vi "OFBS_train_kNN.vi"(6 "Train Data":T4, 8 "error in (no error)":errorcluster, 9 "k":i32, 10 "Parameters":i32[](array[numeric]), 11 "OFBS class in":refnum<class "OptFreqBandsSearch.lvclass">) -> (0 "error out":errorcluster, 1 "Training Results":T2[](array[typedef]) {"Standard Deviation" format="%.2f"}, 2 "Classifier Session (out)":T3, 3 "OFBS class out":refnum<class "OptFreqBandsSearch.lvclass">)   [LabVIEW 2016, in "Optimal Frequency Bands Search.lvlib" / "OptFreqBandsSearch.lvclass"]
doc: "Метод, реализующий построение классификатора на основе многослойного персептрона. Для обучения классификатора используются обучающие данные."
uses:
  OptFreqBandsSearch.lvclass
  OFBS_DataTypes.ctl
  <vilib>/vision/Classification.llb/IMAQ Classifier Session.ctl
  <vilib>/vision/Classification.llb/IMAQ Classifier Nearest Neighbor Training Results.ctl
  <vilib>/vision/Classification.llb/IMAQ Classifier Nearest Neighbor options.ctl
  OptFreqBandsSearch.lvclass/OptFreqBandsSearch.ctl
  Optimal Frequency Bands Search.lvlib
  <vilib>/vision/NI_Vision_Development_Module.lvlib
panel:
  in  "Nearest Neighbor Options":T1={"Method"=1, "Metric"=2, "k"=3} {"Method" items=["Nearest Neighbor", "K Nearest Neighbor", "Minimum Mean Distance"]; "Metric" items=["Maximum", "Sum", "Euclidean"]; "k" min=3}
  # "This VI is a part of BCI Design library, http://www.ru-bci.org \nCopyright © 2020, Sotnikov Peter, All rights reserved. License: CC BY-NC 4.0"
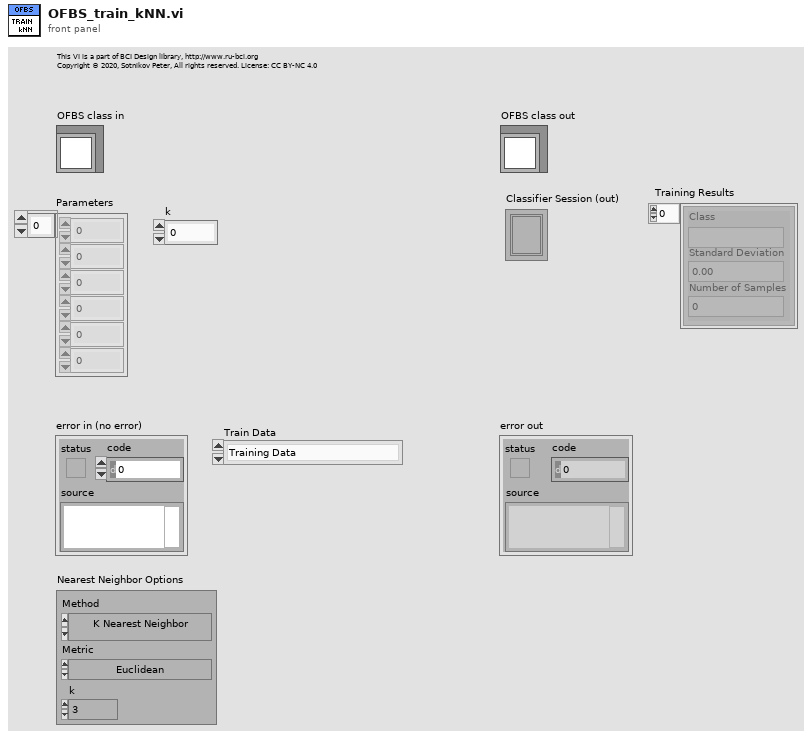
[diagram p1: front panel]
types:
  T1 = typedef "IMAQ Classifier Nearest Neighbor options.ctl" = cluster{"Method":i32, "Metric":i32, "k":i32}
  T2 = typedef "IMAQ Classifier Nearest Neighbor Training Results.ctl" = cluster{"Class":string, "Standard Deviation":sgl, "Number of Samples":i32}
  T3 = typedef "IMAQ Classifier Session.ctl" = refnum<k1>
  T4 = typedef "Optimal Frequency Bands Search.lvlib/OFBS_DataTypes.ctl" = enum16{"Training Data", "Test Data", "Training Data (cross-check)", "Test Data (cross-check)"}
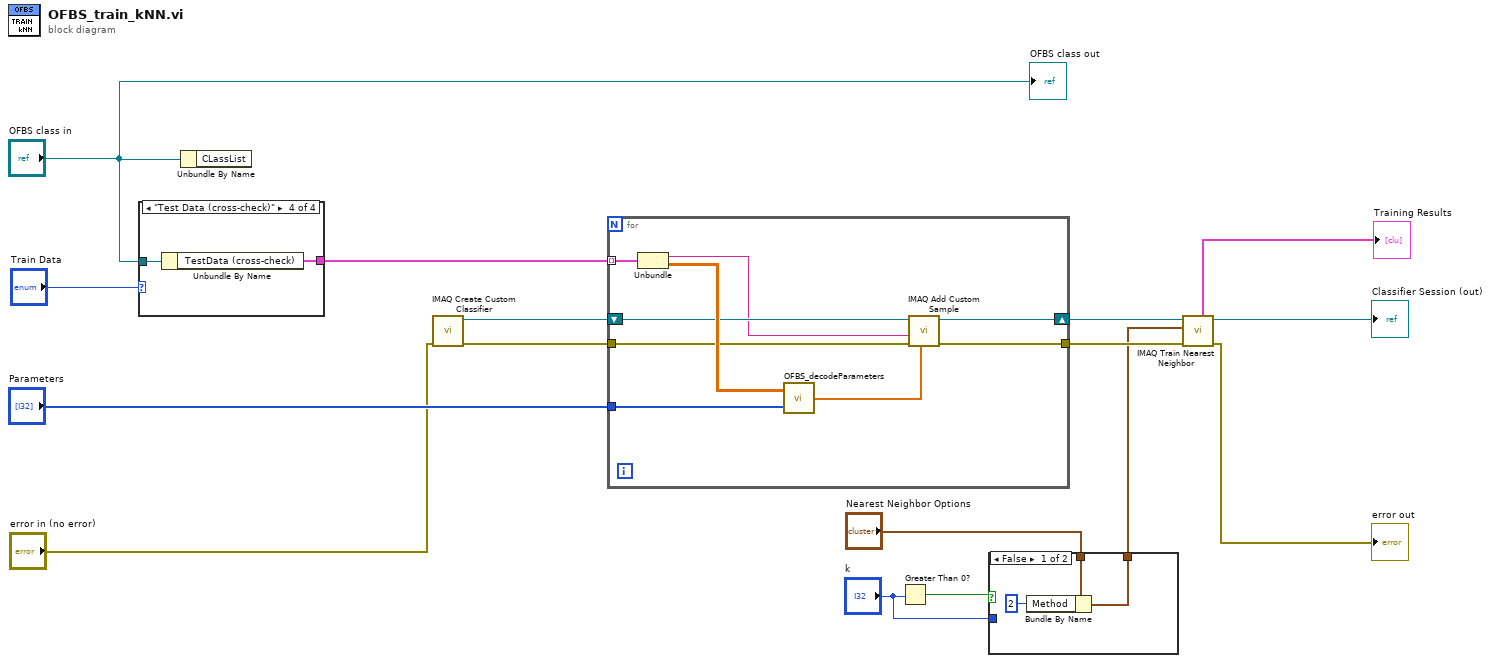
[diagram p0: block diagram]
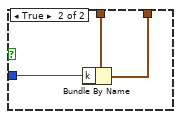
[diagram p2: hidden frame]
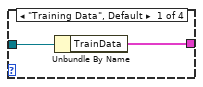
[diagram p3: hidden frame]
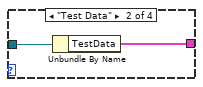
[diagram p4: hidden frame]
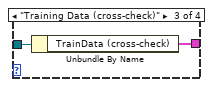
[diagram p5: hidden frame]
diagram:
  n1 = case shown="\"Test Data (cross-check)\"" "Train Data" {
    tunnel: "OFBS class in" -> [w18 w20 w22 w24]
    tunnel: [w17 w19 w21 w23] -> w13
    frame "Training Data", Default {
      n2 = Unbundle By Name(w18) -> ("TrainData"=w17:cluster{"ClassLabel":string, "Trial":dbl[][]}[])
    }
    frame "Test Data" {
      n3 = Unbundle By Name(w20) -> ("TestData"=w19:cluster{"ClassLabel":string, "Trial":dbl[][]}[])
    }
    frame "Training Data (cross-check)" {
      n4 = Unbundle By Name(w22) -> ("TrainData (cross-check)"=w21:cluster{"ClassLabel":string, "Trial":dbl[][]}[])
    }
    frame "Test Data (cross-check)" {
      n5 = Unbundle By Name(w24) -> ("TestData (cross-check)"=w23:cluster{"ClassLabel":string, "Trial":dbl[][]}[])
    }
  }
  n6 = Unbundle By Name("OFBS class in") -> ()  [unwired: 1 out]
  n7 = call "IMAQ Create Custom Classifier"("error in (no error)"="error in (no error)") -> ("error out"=w9:errorcluster, "Classifier Session"=w12:T3)  [unwired: 9 in]
  n8 = for {
    tunnel: w13 -> [w33] mode=indexing
    tunnel: "Parameters" -> [w31]
    shift-right: [w29] -> w11
    shift-left: w12 -> [w30]
    tunnel: w9 -> [w26]
    tunnel: [w25] -> w8
    n9 = Unbundle(w33) -> ("ClassLabel"=w27:string, "Trial"=w32:dbl[][])
    n10 = call "OFBS_decodeParameters.vi"("Parameters"=w31, "Trial"=w32) -> ("FeatureVector"=w28:dbl[])
    n11 = call "IMAQ Add Custom Sample"("Feature Vector"=w28, "error in (no error)"=w26, "Class"=w27, "Classifier Session"=w30) -> ("error out"=w25:errorcluster, "Classifier Session (dup)"=w29:T3)  [unwired: 6 in]
  }
  n12 = Greater Than 0?(x="k") -> (x > 0?=w2:bool)
  n13 = case shown="False" w2 {
    tunnel: "Nearest Neighbor Options" -> [w36 w39]
    tunnel: [w35 w38] -> w3
    tunnel: "k" -> [_ w37]
    frame False {
      n14 = Bundle By Name(cluster=w36, "Method"=2) -> (w35:T1)
    }
    frame True {
      n15 = Bundle By Name(cluster=w39, "k"=w37) -> (w38:T1)
    }
  }
  n16 = call "IMAQ Train Nearest Neighbor"("error in (no error)"=w8, "Nearest Neighbor Options"=w3, "Classifier Session"=w11) -> ("error out"=→"error out":errorcluster, "Classifier Session (dup)"=→"Classifier Session (out)":T3, "Training Results"=→"Training Results":T2[])  [unwired: 5 in, 1 out]
  "OFBS class out" <- "OFBS class in"
